vi "Return_EnFlo_Tunnel_to_Neutral.vi"(3 "Mode":T5, 5 "Traverse line In":T2 {"Carrier_2 Q (l/min)" format="%#.2f"; "Row Duration (mins)" format="%#.1f"; "Row No" min=0; "Trace Gas Concentration (%)" min=0.0 format="%#_4f"; "Carrier_1 Q (l/min)" format="%#.4f"; "Start X" format="%#.2f"; "Start Y" format="%#.2f"; "Start Z" format="%#.2f"; "End X" format="%#.2f"; "End Y" format="%#.2f"; "End Z" format="%#.2f"; "Tunnel Speed" format="%#.2f"; "Averaging time (mins)" min=0.0 format="%#.2f"}) -> (0 "Error Message":string, 1 "Status":T1, 2 "Traverse line Out":T2 {"Carrier_2 Q (l/min)" format="%#.2f"; "Row Duration (mins)" format="%#.1f"; "Row No" min=0; "Trace Gas Concentration (%)" min=0.0 format="%#_4f"; "Carrier_1 Q (l/min)" format="%#.4f"; "Start X" format="%#.2f"; "Start Y" format="%#.2f"; "Start Z" format="%#.2f"; "End X" format="%#.2f"; "End Y" format="%#.2f"; "End Z" format="%#.2f"; "Tunnel Speed" format="%#.2f"; "Averaging time (mins)" min=0.0 format="%#.2f"})   [LabVIEW 2020]
uses:
  ADAM Client/Sub VIs/ADAM Controls/Update_scan_value.ctl
  Gen Trav/Multi_Run_Status.ctl
  ADAM Client/Sub VIs/ADAM Controls/Client_Source_Status.ctl
  Controls/User_Specific_mode.ctl
  Globals/Trav_pos_global.vi
  ADAM Client/Sub VIs/ADAM Controls/Channel_names.ctl
  Controls/GMU Gas Line Name.ctl
  Gen Trav/Spacing.ctl
  Gen Trav/Traverse_cluster.ctl
  Controls/Multi_run_mode.ctl
panel:
  in  "Stop waiting":bool
  out "Chilled water supply temp":dbl(graph)
  # "X           Y          Z"
  # "Start"
  # "End"
  # "X           Y          Z"
  # "Start"
  # "End"
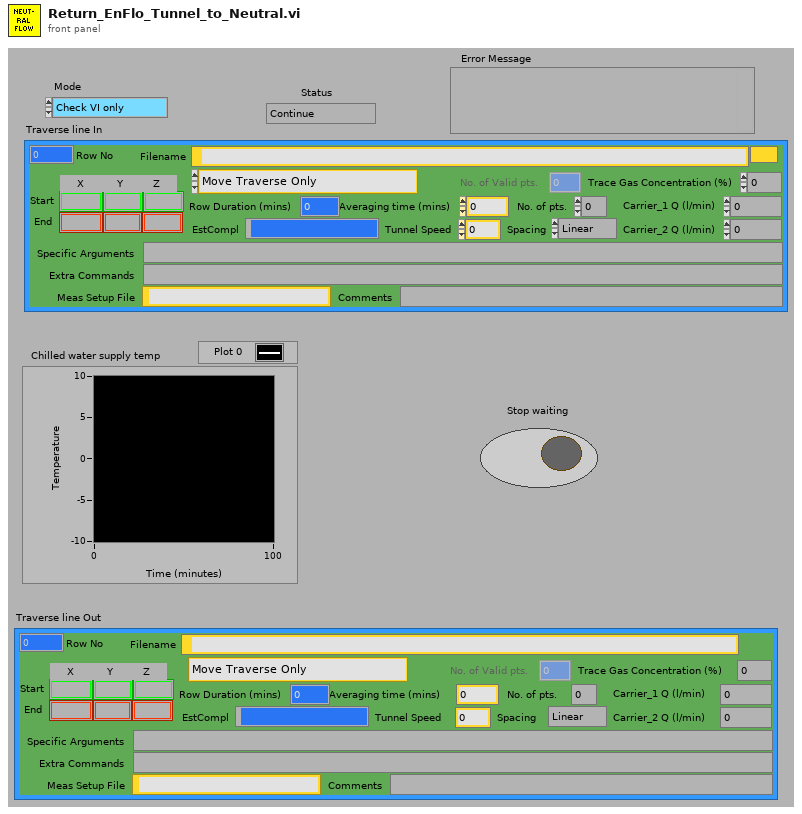
[diagram p1: front panel]
types:
  T1 = typedef "Multi_Run_Status.ctl" = enum16{"Continue", "Continue with Error", "Jump to Next Point", "Jump to Next Row", "Jump To Fall Back", "Terminate Run"}
  T2 = typedef "Traverse_cluster.ctl" = cluster{"Start X":sgl, "Start Y":sgl, "Start Z":sgl, "End X":sgl, "End Y":sgl, "End Z":sgl, "No. of pts.":i32, "Spacing":T3, "Filename":path, "Tunnel Speed":dbl, "Averaging time (mins)":dbl, "Extra Commands":string, "Carrier_1 Q (l/min)":dbl, "Carrier_2 Q (l/min)":dbl, "Trace Gas Concentration (%)":dbl, "Specific Arguments":string, "Comments":string, "Row No":i32, "Row Type Selector":T4, "EstCompl":string, "Row Duration (mins)":dbl, "No. of Valid pts.":i32, "Meas Setup File":string}
  T3 = typedef "Spacing.ctl" = enum16{"Linear", "Log", "Gauss", "Specified", "N/A"}
  T4 = typedef "Multi_run_mode.ctl" = enum16{"Move Traverse Only", "Set Tunnel Speed Only", "Set Source Only", "Set Measurement Conditions", "Single Measurement", "Vertical Profile", "Lateral Profile", "Longitudinal Profile", "Multi-Axis Profile", "Explore Volume", "Auto Calibrate", "Meas Fast FID Bkgnd", "Check Beam Power", "Scanning Valve Measurement", "Run VI Named:", "Set ADAM Ch", "Wait (minutes)", "Send Message", "Synchronize With:", "Fall Back to this Row", "Turn Off Row Repeating", "Traverse 3D Volume", "Blank Row", "Jump to Fall Back Row"}
  T5 = typedef "User_Specific_mode.ctl" = enum16{"Check VI only", "Run VI"}
  T6 = typedef "Update_scan_value.ctl" = cluster{"Channel Name":string, "New Value":dbl}
  T7 = typedef "Channel_names.ctl" = enum16{"Active Only", "Active + Off", "All Channels"}
  T8 = typedef "GMU Gas Line Name.ctl" = enum16{"GMU1 Source", "GMU2 Source", "GMU2 Calib"}
  T9 = typedef "Client_Source_Status.ctl" = enum16{"Not Using", "Using", "Must Have"}
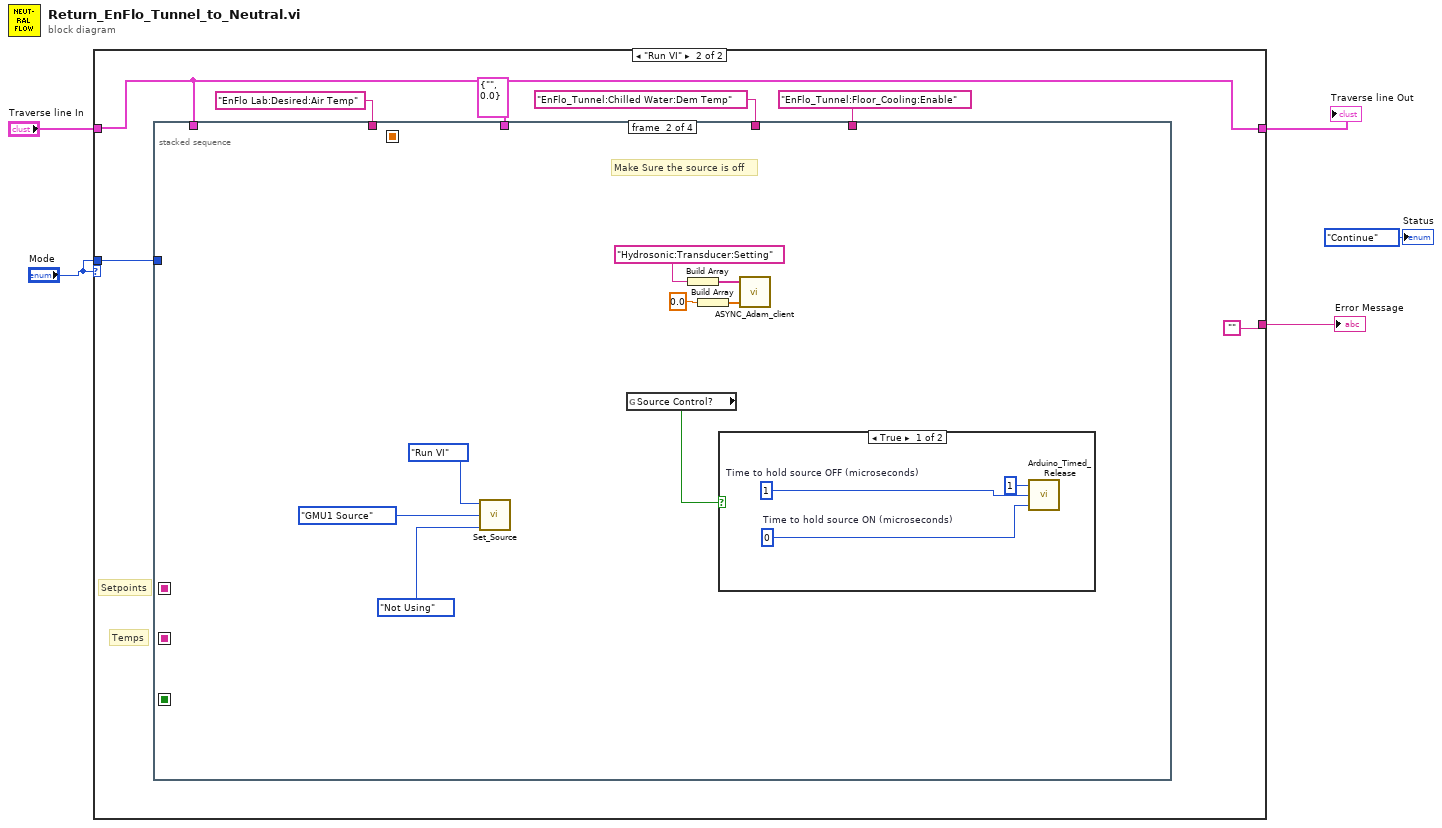
[diagram p0: block diagram]
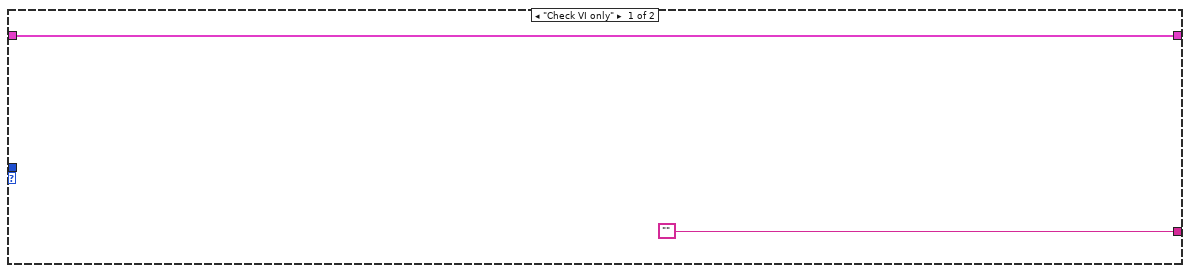
[diagram p2: hidden frame]
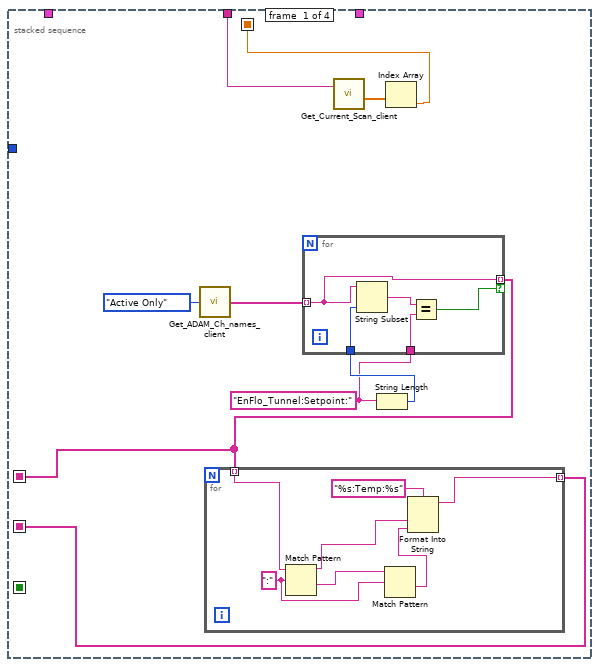
[diagram p3: hidden frame]
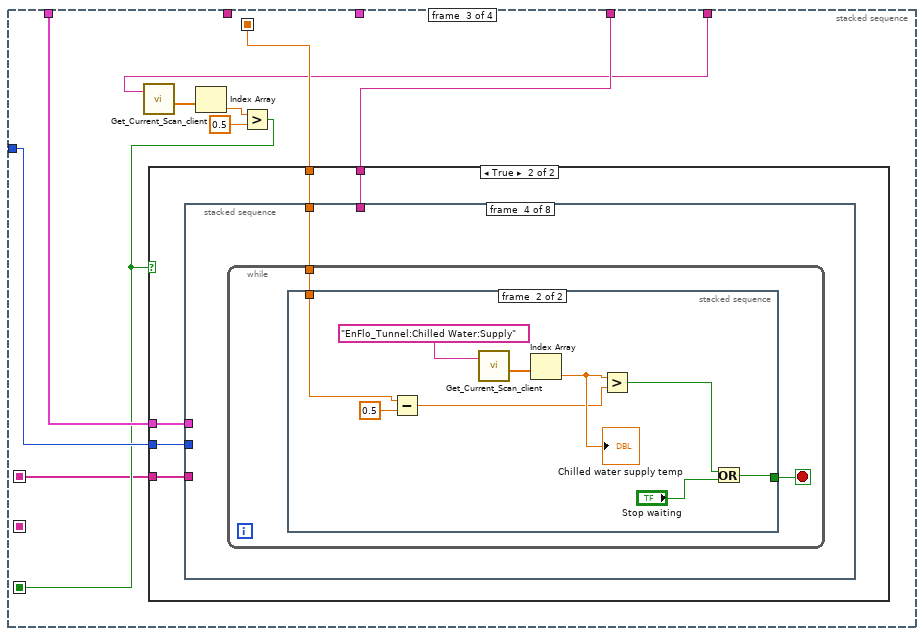
[diagram p5: hidden frame]
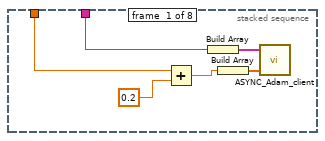
[diagram p7: hidden frame]
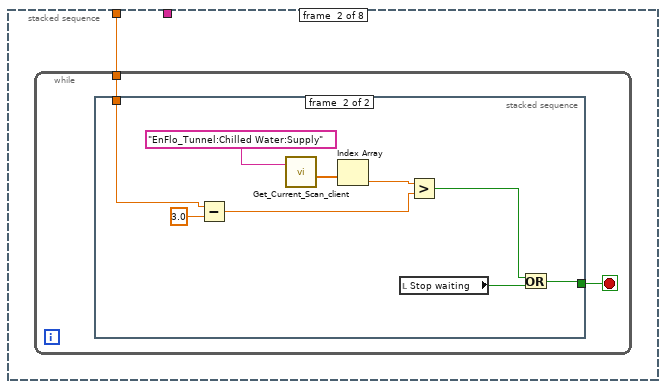
[diagram p8: hidden frame]
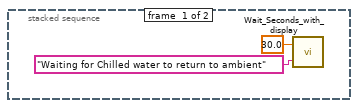
[diagram p9: hidden frame]
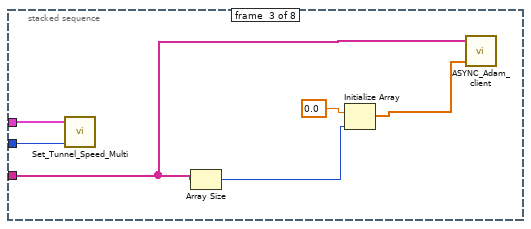
[diagram p10: hidden frame]
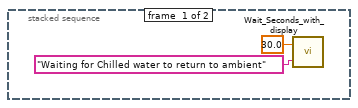
[diagram p11: hidden frame]
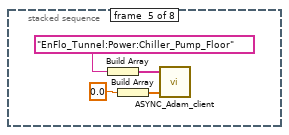
[diagram p12: hidden frame]
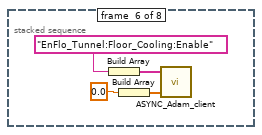
[diagram p13: hidden frame]
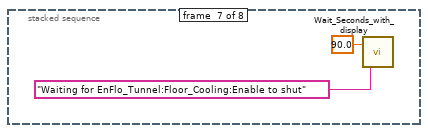
[diagram p14: hidden frame]
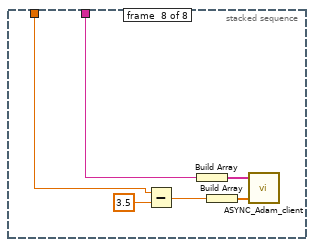
[diagram p15: hidden frame]
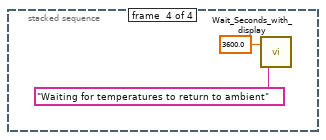
[diagram p16: hidden frame]
diagram:
  n1 = case shown="\"Run VI\"" "Mode" {
    tunnel: "Traverse line In" -> [w7 w12]
    tunnel: [w7 w12] -> w4
    tunnel: ["" ""] -> w3
    tunnel: "Mode" -> [_ w11]
    frame "Check VI only" {
    }
    frame "Run VI" {
      # "Setpoints"
      # "Temps"
      n2 = stacked-sequence {
        seq-local: [w18 _ _ _] -> [_ _ _ _]
        seq-local: [w16 _ _ _] -> [_ _ w55 _]
        seq-local: [_ _ w49 _] -> [_ _ _ _]
        seq-local: [w17 _ _ _] -> [_ _ w48 _]
        tunnel: T6 {"Channel Name"="", "New Value"=0.0} ("Update Scan Value Cluster") -> [_ _ _ _]
        tunnel: w12 -> [_ _ w54 _]
        tunnel: w11 -> [_ _ w53 _]
        tunnel: "EnFlo Lab:Desired:Air Temp" -> [w15 _ _ _]
        tunnel: "EnFlo_Tunnel:Chilled Water:Dem Temp" -> [_ _ w56 _]
        tunnel: "EnFlo_Tunnel:Floor_Cooling:Enable" -> [_ _ w47 _]
        frame #0 {
          w20 = "EnFlo_Tunnel:Setpoint:"
          n3 = call "Get_ADAM_Ch_names_client.vi"("Channel names set"=Channel_names."Active Only") -> ("Ch names"=w19:string[])
          n4 = call "Get_Current_Scan_client.vi"("singleChannel"=w15) -> ("Numerical Values"=w23:dbl[])  [unwired: 1 in, 3 out]
          n5 = String Length(string=w20) -> (length=w21:i32)
          n6 = for {
            tunnel: w19 -> [w32] mode=indexing
            tunnel: w21 -> [w35]
            tunnel: w20 -> [w34]
            tunnel: [w32] -> w17 mode=indexing if=w31
            n7 = String Subset(string=w32, length (rest)=w35) -> (substring=w33:string)  [unwired: 1 out]
            n8 = Equal?(x=w33, y=w34) -> (x = y?=w31:bool)
          }
          n9 = for {
            tunnel: w17 -> [w24] mode=indexing
            tunnel: [w25] -> w18 mode=indexing
            w29 = ":" ("regular expression")
            n10 = Match Pattern(string=w24, regular expression=w29) -> (before substring=w27:string, after substring=w30:string)  [unwired: 3 out]
            n11 = Match Pattern(string=w30, regular expression=w29) -> (after substring=w26:string)  [unwired: 4 out]
            n12 = Format Into String(format string="%s:Temp:%s", w27, w26) -> (resulting string=w25:string)  [unwired: 2 in, 1 out]
          }
          n13 = Index Array(array=w23) -> (element=w16:dbl)  [unwired: 1 in]
        }
        frame #1 {
          # "Make Sure the source is off"
          n14 = call "Set_Source.vi"("Source Status"=Client_Source_Status."Not Using", "Gas Line Name"=GMU_Gas_Line_Name."GMU1 Source", "Simulate/Run"=User_Specific_mode."Run VI") -> ()  [unwired: 1 in, 6 out]
          n15 = global read "Trav_pos_global.vi" "Source Control?"() -> (w41:bool)
          n16 = Build Array("Hydrosonic:Transducer:Setting") -> (w38:string[])
          n17 = Build Array(0.0 ("element")) -> (w39:dbl[])
          n18 = case shown="True" w41 {
            frame True {
              w45 = u32 1  # Time to hold source OFF (microseconds)
              w44 = u32 0  # Time to hold source ON (microseconds)
              n19 = call "Arduino_Timed_Release.vi"("Time to hold source ON (microseconds)"=w44, "Time to hold source OFF (microseconds)"=w45, "Number of cycles"=u16 1) -> ()  [unwired: 2 out]
            }
            frame False {
            }
          }
          n20 = call "ASYNC_Adam_client.vi"("Values"=w39, "Channel Names"=w38) -> ()  [unwired: 1 in, 2 out]
        }
        frame #2 {
          n21 = call "Get_Current_Scan_client.vi"("singleChannel"=w47) -> ("Numerical Values"=w52:dbl[])  [unwired: 1 in, 3 out]
          n22 = Index Array(array=w52) -> (element=w51:dbl)  [unwired: 1 in]
          n23 = Greater?(x=w51, y=0.5) -> (0:w49:bool)
          n24 = case shown="True" w49 {
            tunnel: w56 -> [_ w58]
            tunnel: w55 -> [_ w59]
            tunnel: w54 -> [_ w61]
            tunnel: w53 -> [_ w60]
            tunnel: w48 -> [_ w57]
            frame False {
            }
            frame True {
              n25 = stacked-sequence {
                tunnel: w61 -> [_ _ w83 _ _ _ _ _]
                tunnel: w60 -> [_ _ w82 _ _ _ _ _]
                tunnel: w59 -> [w64 w68 _ w88 _ _ _ w112]
                tunnel: w58 -> [w65 _ _ _ _ _ _ w113]
                tunnel: w57 -> [_ _ w84 _ _ _ _ _]
                frame #0 {
                  n26 = Add(x=w64, y=0.2) -> (x+y=w63:dbl)
                  n27 = Build Array(w65) -> (w66:string[])
                  n28 = Build Array(w63) -> (w67:dbl[])
                  n29 = call "ASYNC_Adam_client.vi"("Values"=w67, "Channel Names"=w66) -> ()  [unwired: 1 in, 2 out]
                }
                frame #1 {
                  n30 = while {
                    tunnel: w68 -> [w69]
                    stop <- w70 stop-if-true
                    n31 = stacked-sequence {
                      tunnel: [_ w78] -> w70
                      tunnel: w69 -> [_ w77]
                      frame #0 {
                        n32 = call "Wait_Seconds_with_display.vi"("Message"="Waiting for Chilled water to return to ambient", "Seconds to wait"=30.0) -> ()  [unwired: 1 in, 1 out]
                      }
                      frame #1 {
                        n33 = Subtract(x=w77, y=3.0) -> (x-y=w75:dbl)
                        n34 = call "Get_Current_Scan_client.vi"("singleChannel"="EnFlo_Tunnel:Chilled Water:Supply") -> ("Numerical Values"=w81:dbl[])  [unwired: 1 in, 3 out]
                        n35 = Index Array(array=w81) -> (element=w80:dbl)  [unwired: 1 in]
                        n36 = local read "Stop waiting"() -> (w74:bool)
                        n37 = Greater?(x=w80, y=w75) -> (0:w79:bool)
                        n38 = Or(x=w79, y=w74) -> (x .or. y?=w78:bool)
                      }
                    }
                  }
                }
                frame #2 {
                  n39 = call "Set_Tunnel_Speed_Multi.vi"("Simulate/Run"=w82, "Traverse line"=w83) -> ()  [unwired: 4 out]
                  n40 = Array Size(array=w84) -> (size(s)=w87:i32)
                  n41 = Initialize Array(0.0 ("Input Element"), w87) -> (w85:dbl[])
                  n42 = call "ASYNC_Adam_client.vi"("Values"=w85, "Channel Names"=w84) -> ()  [unwired: 1 in, 2 out]
                }
                frame #3 {
                  n43 = while {
                    tunnel: w88 -> [w89]
                    stop <- w90 stop-if-true
                    n44 = stacked-sequence {
                      tunnel: [_ w98] -> w90
                      tunnel: w89 -> [_ w96]
                      frame #0 {
                        n45 = call "Wait_Seconds_with_display.vi"("Message"="Waiting for Chilled water to return to ambient", "Seconds to wait"=30.0) -> ()  [unwired: 1 in, 1 out]
                      }
                      frame #1 {
                        n46 = Subtract(x=w96, y=0.5) -> (x-y=w94:dbl)
                        n47 = call "Get_Current_Scan_client.vi"("singleChannel"="EnFlo_Tunnel:Chilled Water:Supply") -> ("Numerical Values"=w101:dbl[])  [unwired: 1 in, 3 out]
                        n48 = Index Array(array=w101) -> (element=w100:dbl)  [unwired: 1 in]
                        "Chilled water supply temp" <- w100
                        n49 = Greater?(x=w100, y=w94) -> (0:w99:bool)
                        n50 = Or(x=w99, y="Stop waiting") -> (x .or. y?=w98:bool)
                      }
                    }
                  }
                }
                frame #4 {
                  n51 = Build Array("EnFlo_Tunnel:Power:Chiller_Pump_Floor") -> (w104:string[])
                  n52 = Build Array(0.0 ("element")) -> (w103:dbl[])
                  n53 = call "ASYNC_Adam_client.vi"("Values"=w103, "Channel Names"=w104) -> ()  [unwired: 1 in, 2 out]
                }
                frame #5 {
                  n54 = Build Array("EnFlo_Tunnel:Floor_Cooling:Enable") -> (w107:string[])
                  n55 = Build Array(0.0 ("element")) -> (w108:dbl[])
                  n56 = call "ASYNC_Adam_client.vi"("Values"=w108, "Channel Names"=w107) -> ()  [unwired: 1 in, 2 out]
                }
                frame #6 {
                  n57 = call "Wait_Seconds_with_display.vi"("Message"="Waiting for EnFlo_Tunnel:Floor_Cooling:Enable to shut", "Seconds to wait"=90.0) -> ()  [unwired: 1 in, 1 out]
                }
                frame #7 {
                  n58 = Subtract(x=w112, y=3.5) -> (x-y=w114:dbl)
                  n59 = Build Array(w113) -> (w117:string[])
                  n60 = Build Array(w114) -> (w116:dbl[])
                  n61 = call "ASYNC_Adam_client.vi"("Values"=w116, "Channel Names"=w117) -> ()  [unwired: 1 in, 2 out]
                }
              }
            }
          }
        }
        frame #3 {
          n62 = call "Wait_Seconds_with_display.vi"("Message"="Waiting for temperatures to return to ambient", "Seconds to wait"=3600.0) -> ()  [unwired: 1 in, 1 out]
        }
      }
    }
  }
  "Traverse line Out" <- w4
  "Error Message" <- w3
  "Status" <- Multi_Run_Status."Continue" ("Status")
